vi "04-QNET_MECHKIT_Potentiometer.vi"() -> ()   [LabVIEW 2012]
doc: "This VI is to be used with the NI-ELVIS and the QNET-Mechatronic Sensors I module. The objective is to calibrate the potentiometer."
uses:
  <vilib>/Simulation/Scripting/Companion Diagram/SimConfigNode/SimParams.ctl
  <vilib>/Simulation/Scripting/Companion Diagram/SimConfigNode/_simSolvers.ctl
  <vilib>/Simulation/Implementation/Shared/SIMSCR Execution Mode.ctl
  <vilib>/Simulation/Param Hierarchy/Typedefs/SIMPH Param Control Actions.ctl
  <vilib>/Simulation/Implementation/Shared/NILVSim_ParamChanged.vi
  <vilib>/Simulation/SignalDisplay/Implementation/NILVSim Time Waveform.llb/SIM Time Waveform (scalar).vi
  <vilib>/Simulation/Utility/Implementation/SIM Halt.vi
  <vilib>/Simulation/Implementation/Shared/NILVSim_Manager.vi
  <vilib>/Simulation/Implementation/Shared/NILVSim_FinalizeModel.vi
  <vilib>/Simulation/Implementation/Shared/SIM Unbundle Sim Info.vi
  <vilib>/Utility/error.llb/Clear Errors.vi
  <vilib>/Simulation/Implementation/Shared/NILVSim_GetModelError.vi
  <vilib>/Simulation/Implementation/Shared/SIM Bundle Sim Info.vi
  <vilib>/Simulation/Implementation/Shared/SIMSH Read Queue.vi
  <vilib>/Simulation/Implementation/Shared/NILVSim_Initialize.vi
  <vilib>/Analysis/6fits.llb/Linear Fit.vi
  <vilib>/DAQmx/read.llb/DAQmx Read.vi
  <vilib>/DAQmx/read.llb/DAQmx Read (Analog DBL 1Chan 1Samp).vi
  <vilib>/Simulation/Utility/Implementation/NILVSim Get Time and IsAcceptedStep.vi
  <vilib>/Simulation/Scripting/Companion Diagram/SimConfigNode/SimDog.xnode
  <vilib>/Simulation/Implementation/XNodeFramework/SimXNode/SimX.xnode
  <vilib>/Analysis/NI_AALPro.lvlib
  <vilib>/Simulation/Implementation/Shared/NI_SIM_Implementation.lvlib
panel:
  in  "Sampling Rate (Hz)":dbl=100.0 min=0.0 max=1000.0 step=25.0 format="%.1f"
  in  "Device":tag="Dev1"
  in  "Tab Control":enum32{"Collect Data", "Calibrate Sensor"}(tab)
  out "slope":dbl format="%_3f"
  out "intercept":dbl format="%_3f"
  out "Potentiometer (V)":waveform(dbl)(graph)
  in  "Pot Angle (deg)":dbl[](array[numeric])
  in  "Sensor Measurement (V)":dbl[](array[numeric])
  out "Sensor Readings":T1(graph)
  out "Display: Potentiometer (deg)":dbl(knob) scale format="%_3f"
  in  "Offset (deg)":dbl
  in  "Calibration Gain (deg/V)":dbl
  out "Potentiometer (deg)":waveform(dbl)(graph)
  in  "stop":bool
  # "QNET-MECHKIT Potentiometer"
  # "NOTE: Place J10 jumper on \"Potentiometer\" setting."
  # "1) Rotate onboard potentiometer to certain position. Enter it in \"Pot Angle (deg)\" array.\n2) Enter corresponding measured sensor voltage in \"Sensor Voltage (V)\" array.\n3) Fill out table with appropriate amount of data points."
  # "Linear curve fitting results:"
  # "Enter gain and offset values for potentiometer to measure correct angle \n(e.g. when pot arrow turned to 45.0 deg, indicators below should read 45.0 deg)."
  # "y = Gain*x + Offset\nwhere\nx is the sensor voltage \ny is the output in centimeters."
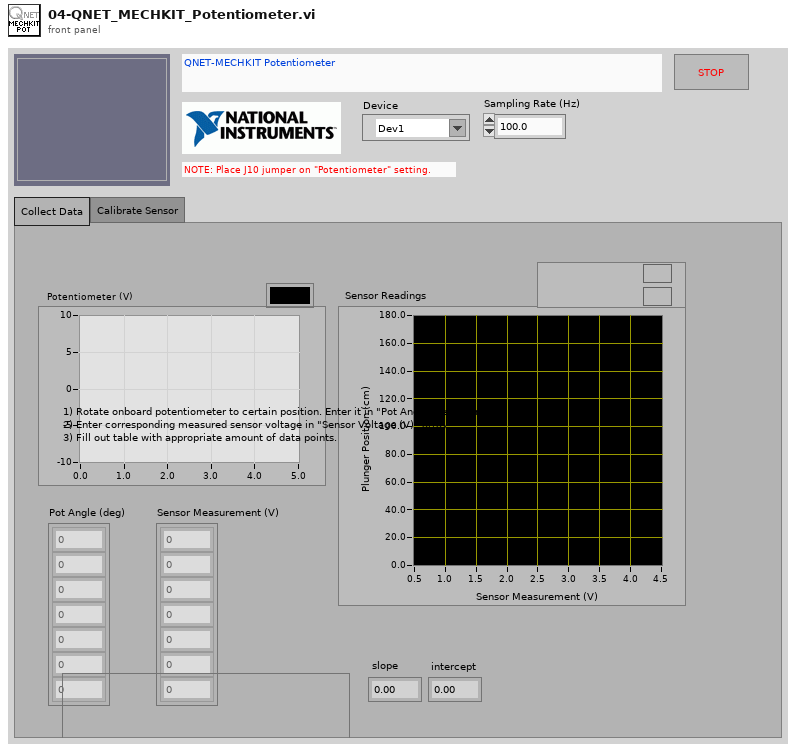
[diagram p1: front panel]
types:
  T1 = cluster{"Sensor Measurement (V)":dbl[], "Best Linear Fit":dbl[]}[]
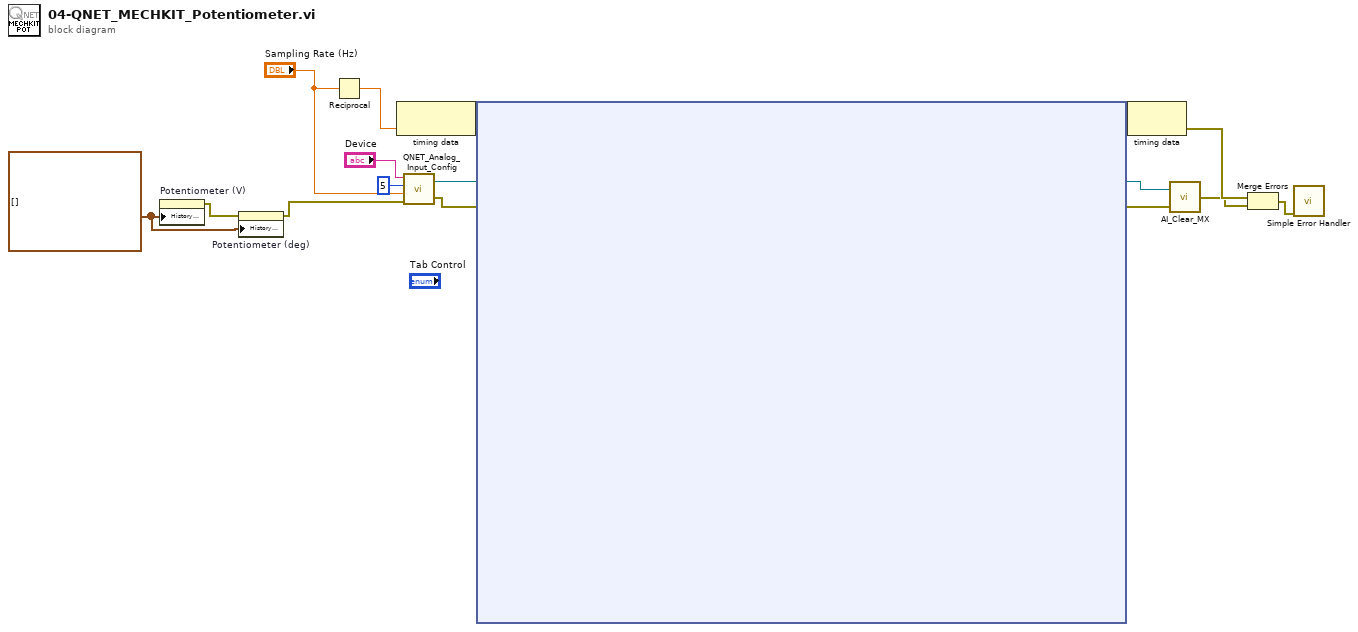
[diagram p0: block diagram]
diagram:
  w1 = waveform(dbl)[] [] ("History Data")
  n1 = property on="Potentiometer (V)" class="WFChart (strict)"("History Data"=w1) -> (error out=w3:errorcluster)  [unwired: 2 in, 1 out]
  n2 = property on="Potentiometer (deg)" class="WFChart (strict)"(error in=w3, "History Data"=w1) -> (error out=w2:errorcluster)  [unwired: 1 in, 1 out]
  n3 = Reciprocal(x="Sampling Rate (Hz)") -> (1/x=w8:dbl)
  n4 = node-c288(w8) -> (w16:variant)
  n5 = call "QNET_Analog_Input_Config.vi"("error in"=w2, "sampling rate (Hz)"="Sampling Rate (Hz)", "analog input channel"=u32 5, "dev"="Device") -> ("error out"=w13:errorcluster, "task out"=w12:refnum<k21>)
  n6 = node-c254 ("Simulation Loop")(w16, w13, w12) -> (w15:variant, w11:refnum<k21>, w10:errorcluster)
  n7 = node-c288(w15) -> (w7:errorcluster)
  n8 = call "AI_Clear_MX.vi"("Error in"=w10, "Task in"=w11) -> ("Error out"=w6:errorcluster)
  n9 = Merge Errors(w7, w6) -> (w5:errorcluster)
  n10 = call <vilib>:"Simple Error Handler.vi"("error in (no error)"=w5) -> ()  [unwired: 1 in, 8 out]
